vi "Pix2Pos.vi"(8 "error in":errorcluster, 9 "Diamètre balle":i32, 10 "Billard rect":T1, 11 "path fichier":path) -> (0 "error out":errorcluster, 2 "Return code C":i32, 3 "Stderr du C":string)   [LabVIEW 2025]
panel:
  out "Command line":string
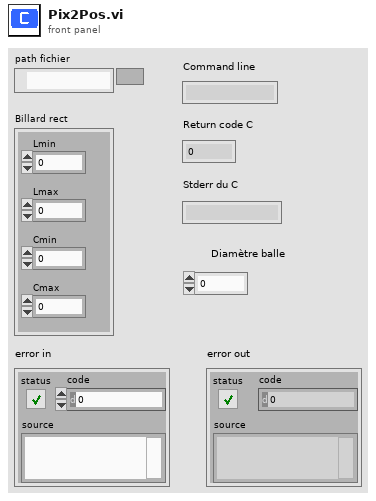
[diagram p1: front panel]
types:
  T1 = cluster{"Lmin":i32, "Lmax":i32, "Cmin":i32, "Cmax":i32}
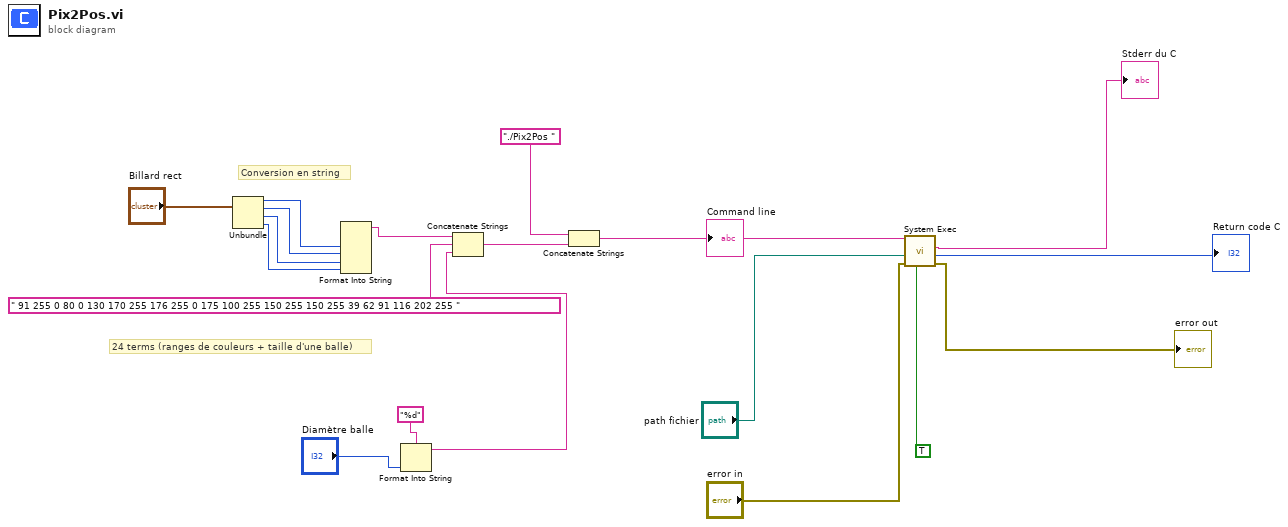
[diagram p0: block diagram]
diagram:
  # "24 terms (ranges de couleurs + taille d'une balle)"
  # "Conversion en string"
  n1 = Unbundle("Billard rect") -> ("Lmin"=w18:i32, "Lmax"=w17:i32, "Cmin"=w16:i32, "Cmax"=w15:i32)
  n2 = Format Into String(w18, w17, w16, w15) -> (resulting string=w14:string)  [unwired: 3 in, 1 out]
  n3 = Format Into String(format string="%d", "Diamètre balle") -> (resulting string=w2:string)  [unwired: 2 in, 1 out]
  n4 = Concatenate Strings(w14, " 91 255 0 80 0 130 170 255 176 255 0 175 100 255 150 255 150 255 39 62 91 116 202 255 ", w2) -> (w12:string)
  n5 = Concatenate Strings("./Pix2Pos ", w12) -> (w10:string)
  "Command line" <- w10
  n6 = call <vilib>:"System Exec.vi"("run minimized? (F)"=TRUE, "error in (no error)"="error in", "working directory"="path fichier", "command line"=w10) -> ("error out"=→"error out":errorcluster, "return code"=→"Return code C":i32, "standard error"=→"Stderr du C":string)  [unwired: 4 in, 1 out]
